vi "UHR-Fleezers Control (host) - 12.5.vi"() -> ()   [LabVIEW 2012] (continued)
    n2798 = xnode ("Read/Write Control")("FPGA VI Reference In"=w3268, "error in"=w3267) -> ("FPGA VI Reference Out"=w3103:T20, "error out"=w3102:errorcluster, "AI2 Y Sum Set 1"=w3366:i16, "AI2 Y Sum Set 2"=w3365:i16, "AI1 X Set 1"=w3167:fxp<+/-,16,1>, "AI1 X Set 2"=w3166:fxp<+/-,16,1>, "Trap Pos FB Int Signal"=→"Trap Pos FB Int Signal":fxp<+/-,24,9>, "Trap Pos FB Int-Norm Signal"=→"Trap Pos FB Int-Norm Signal":fxp<+/-,16,1>, "Trap Pos FB Action"=w3160:i64, "Scanning"=→"AOD Scanning":bool, "Scan I"=→"AOD Scan I":u64, "Scanning MCL"=w3368:bool, "Scan I (MCL)"=→"MCL Scan I":u64, "Green FB Sum"=w3305:i16, "Trap Pos FB Action"=w3090:i64, "TTrig Fin Thresh"=w3086:i64, "Red FB Intensity"=w3067:i16, "Blue Intensity"=w3062:i16)
    "MCL Scanning" <- w3368
    "Trap Pos FB Action" <- w3160
    n2799 = Divide(x=w3067, y=3276.7) -> (x/y=w3066:dbl)
    "Red laser intensity (V)" <- w3066
    n2800 = Divide(x=w3062, y=3276.7) -> (x/y=w3061:dbl)
    "Blue laser intensity (V)" <- w3061
    n2801 = Divide(x=w3305, y=3276.7) -> (x/y=w3065:dbl)
    "Green laser intensity (V)" <- w3065
    n2802 = local read "FB Trig Integrate"() -> (w3084:u32)
    n2803 = Divide(x=w3090, y=w3084) -> (x/y=w3083:dbl)
    "TTrig Sig (Int)" <- w3083
    n2804 = Bundle(w3065, w3066, w3061) -> (→"Fluorescence laser intensities plot":cluster{dbl, dbl, dbl})  [unwired: 1 in]
    n2805 = Divide(x=w3086, y=w3084) -> (x/y=w3081:dbl)
    "TTrig Fin Thresh (Int)" <- w3081
    n2806 = local read "AOM X Cal (nm/MHz)"() -> (w3089:dbl)
    n2807 = local read "AI2 (V)"() -> (w3367:cluster{"Set 1":dbl, "Set 2":dbl})
    n2808 = Bundle By Name(cluster=w3367, "Set 1"=w3366, "Set 2"=w3365) -> (w3363:cluster{"Set 1":dbl, "Set 2":dbl})
    n2809 = Divide(x=w3160, y=327.67) -> (x/y=→"Action (%)":dbl)
    n2810 = local read "Trap X (AI1)"() -> (w3180:T10)
    n2811 = call "IR AOM word double to freq.vi"("Frequency Word In (double)"=w3081) -> ("Frequency Out (MHz)"=w3080:dbl)
    n2812 = call "IR AOM word double to freq.vi"("Frequency Word In (double)"=w3083) -> ("Frequency Out (MHz)"=w3082:dbl)
    n2813 = Divide(x=w3363, y=3276.7) -> (x/y=w3362:cluster{"Set 1":dbl, "Set 2":dbl})
    n2814 = Multiply(x=w3082, y=w3089) -> (x*y=w3088:dbl)
    "TTrig Sig (nm)" <- w3088
    n2815 = Multiply(x=w3080, y=w3089) -> (x*y=w3087:dbl)
    "TTrig Fin Thresh (nm)" <- w3087
    n2816 = local write "AI2 (V)"(w3362) -> ()
    n2817 = Bundle(cluster=w3180, "Trap 1"=w3167, "Trap 2"=w3166) -> (→"Trap X (AI1)":T10)
    n2818 = Bundle(w3088, w3087) -> (→"TTrig":cluster{dbl, dbl})  [unwired: 1 in]
    n2819 = flat-sequence "To save data" {
      tunnel: [w4458] -> w3386
      tunnel: [w4459] -> w3385
      tunnel: w3336 -> [w4452]
      tunnel: w3108 -> [w4456]
      tunnel: ["Save Calibration"] -> w3359
      tunnel: w3356 -> [w4455]
      tunnel: [w4448] -> w3355
      tunnel: [w4445] -> w3354
      tunnel: [w4442] -> w3353
      tunnel: w3335 -> [w4444]
      tunnel: w3250 -> [w4438]
      tunnel: [w4438] -> w3249
      tunnel: ["Start Saving"] -> w3219
      tunnel: [w4432] -> w3148
      tunnel: [w4431] -> w3147
      tunnel: w3386 -> [w4706]
      tunnel: w3385 -> [w4705]
      tunnel: w3149 -> [w4704]
      tunnel: w3359 -> [w4703]
      tunnel: w3355 -> [w4701]
      tunnel: w3354 -> [w4700]
      tunnel: w3353 -> [w4699]
      tunnel: w3228 -> [w4698]
      tunnel: w3260 -> [w4697]
      tunnel: w3249 -> [w4696]
      tunnel: w3219 -> [w4695]
      tunnel: w3217 -> [w4694]
      tunnel: w3045 -> [w4693]
      tunnel: w3148 -> [w4692]
      tunnel: w3147 -> [w4691]
      tunnel: w3146 -> [w4690]
      tunnel: w3069 -> [w4689]
      frame #0 {
        n2820 = Or(x="Save N Sets", y="Start Saving") -> (x .or. y?=w4439:bool)
        n2821 = To Double Precision Float(number=w4455) -> (double precision float=w4449:dbl)
        n2822 = Build Array(w4439, "Save Calibration", w4452, w4444) -> (w4454:bool[])
        n2823 = Compound Arithmetic op=OR("Save Calibration", w4452, w4439, w4444) -> (w4457:bool)
        n2824 = Boolean Array To Number(Boolean array=w4454) -> (number=w4451:u32)
        n2825 = feedback #27(FALSE ("Save APD Data\nwith Trap Data")) -> (w4433:bool)
        n2826 = feedback #28(refnum<k0> refnum) -> (w4460:refnum<file>)
        n2827 = feedback #29(refnum<k0> refnum) -> (w4435:refnum<file>)
        n2828 = feedback #30(FALSE ("Save APD Data\nwith Trap Data")) -> (w4443:bool)
        n2829 = feedback #31(refnum<k0> refnum) -> (w4446:refnum<file>)
        n2830 = feedback #32(0) -> (w4462:i32)
        n2831 = feedback #33() -> (w4450:u32)  [unwired: 1 out]
        n2832 = case shown="True" w4457 {
          tunnel: [w4469 1] -> w4458
          tunnel: w4462 -> [w4471 _]
          tunnel: [w4470 w4502] -> w4459
          tunnel: w4460 -> [w4470 _]
          tunnel: w4456 -> [_ w4520]
          tunnel: w4449 -> [_ w4518]
          tunnel: w4451 -> [_ w4521]
          tunnel: [w4468 w4501] -> w4448
          tunnel: w4450 -> [w4468 _]
          tunnel: [w4467 w4499] -> w4445
          tunnel: w4446 -> [w4467 _]
          tunnel: [w4466 w4498] -> w4442
          tunnel: w4443 -> [w4466 _]
          tunnel: "Start Saving" -> [_ w4496]
          tunnel: w4438 -> [_ w4495]
          tunnel: [w4465 w4487] -> w4431
          tunnel: w4435 -> [w4465 _]
          tunnel: [w4464 w4486] -> w4432
          tunnel: w4433 -> [w4464 _]
          frame False {
            n2833 = Increment(x=w4471) -> (x+1=w4469:i32)
          }
          frame True {
            w4492 = FALSE ("Start Saving")
            w4497 = 9.0  # File Version
            w4504 = FALSE ("prepend array or string size? (T)")
            w4503 = T27."big-endian, network order" ("byte order (0:big-endian, network order)")
            n2834 = local read "BD 1 Frequency 1 (MHz)"() -> (w4517:dbl)
            n2835 = local read "BD 2 Frequency 1 (MHz)"() -> (w4516:dbl)
            n2836 = local read "BD 1 Frequency 2 (MHz)"() -> (w4515:dbl)
            n2837 = local read "BD 2 Frequency 2 (MHz)"() -> (w4514:dbl)
            n2838 = local read "BD 1 Frequency 3 (MHz)"() -> (w4513:dbl)
            n2839 = local read "BD 2 Frequency 3 (MHz)"() -> (w4512:dbl)
            n2840 = Array Size(array=w4495) -> (size(s)=w4494:i32)
            n2841 = To Double Precision Float(number=w4494) -> (double precision float=w4493:dbl)
            n2842 = local write "Save Calibration"(w4492) -> ()
            n2843 = local write "Start Saving"(w4492) -> ()
            n2844 = Build Array("Save APD Data\nwith Trap Data", "Save Trap Pos. Data") -> (w4489:bool[])
            n2845 = Boolean Array To Number(Boolean array=w4489) -> (number=w4488:u32)
            n2846 = Build Array(w4517, w4516, w4515, w4514, w4513, w4512) -> (w4511:dbl[])
            n2847 = case shown="1, Default" w4521 {
              tunnel: w4520 -> [w4593 w4613 w4629 w4667]
              tunnel: w4493 -> [w4598 w4620 w4649 w4686]
              tunnel: w4518 -> [w4597 w4619 w4648 w4685]
              tunnel: [w4594 w4615 w4640 w4677] -> w4509
              tunnel: [w4585 "Cal sets to save" w4630 w4668] -> w4501
              tunnel: w4511 -> [w4595 w4616 w4642 w4679]
              tunnel: "Save APD Data\nwith Trap Data" -> [w4592 _ w4626 w4665]
              tunnel: [w4592 w4607 w4626 w4665] -> w4498
              tunnel: w4497 -> [w4588 w4608 w4624 w4663]
              tunnel: w4496 -> [w4587 _ _ _]
              tunnel: [w4578 w4607 w4623 w4653] -> w4486
              tunnel: "Save Trap Pos. Data" -> [w4578 _ w4623 w4653]
              tunnel: w4488 -> [w4577 _ w4622 w4652]
              frame 1, Default {
                # "timeseries"
                n2848 = case shown="True" "Profile" {
                  tunnel: [w4601 w4605] -> w4582
                  tunnel: [w4601 w4604] -> w4581
                  tunnel: [w4601 w4603] -> w4580
                  tunnel: [w4601 w4602] -> w4579
                  frame False {
                    w4601 = 0.0 ("f")
                  }
                  frame True {
                    n2849 = local read "Current Position"() -> (w4606:cluster{dbl, dbl, dbl})
                    n2850 = local read "Y change (mm)"() -> (w4602:dbl)
                    n2851 = Unbundle(w4606) -> (w4605:dbl, w4604:dbl, w4603:dbl)
                  }
                }
                n2852 = local read "Save ave N"() -> (w4600:dbl)
                n2853 = Multiply(x=w4600, y=w4593) -> (x*y=w4599:dbl)
                n2854 = To Double Precision Float(number=w4577) -> (double precision float=w4591:dbl)
                n2855 = Build Array(w4588, w4593, w4599, w4598, w4597, 0.0 ("f")) -> (w4596:dbl[])
                n2856 = Build Array(w4591, w4582, w4581, w4580, w4579) -> (w4589:dbl[])
                n2857 = Select(t=u32 4000000000, s=w4587, f="N sets to save") -> (s? t:f=w4585:u32)
                n2858 = Build Array (concatenate)(w4596, w4595, w4589) -> (w4594:dbl[])
              }
              frame 2 {
                w4610 = 0.0 ("f")
                w4607 = FALSE ("Save APD Data\nwith Trap Data")
                # "calibration"
                n2859 = Boolean To (0,1)(Boolean=w4607) -> (0, 1=w4612:i16)
                n2860 = To Double Precision Float(number=w4612) -> (double precision float=w4611:dbl)
                n2861 = Build Array(w4611, w4610, w4610, w4610, w4610) -> (w4609:dbl[])
                n2862 = Build Array(w4608, w4613, w4613, w4620, w4619, 1.0 ("t")) -> (w4617:dbl[])
                n2863 = Build Array (concatenate)(w4617, w4616, w4609) -> (w4615:dbl[])
                "Calibrating Trap..." <- TRUE ("Calibrating...")
              }
              frame 4 {
                w4627 = 0.0 ("f")
                # "scan dir (x/y = 0/1)"
                # "cycles/step"
                # "n scans (f/b)"
                # "steps"
                # "freq. range"
                # "AOD raster scan"
                n2864 = local read "Number of F/B Scans (AOD)"() -> (w4634:u16)
                n2865 = local read "Cycles/step (AOD)"() -> (w4636:u64)
                n2866 = local read "Scan Range (MHz)"() -> (w4639:dbl)
                n2867 = local read "Scan steps (AOD)"() -> (w4638:u64)
                n2868 = local read "Scan BD"() -> (w4646:bool)
                n2869 = local read "Save ave N"() -> (w4651:dbl)
                n2870 = Boolean To (0,1)(Boolean=w4646) -> (0, 1=w4645:i16)
                n2871 = To Double Precision Float(number=w4634) -> (double precision float=w4633:dbl)
                n2872 = To Double Precision Float(number=w4638) -> (double precision float=w4637:dbl)
                n2873 = To Double Precision Float(number=w4636) -> (double precision float=w4635:dbl)
                n2874 = To Double Precision Float(number=w4645) -> (double precision float=w4644:dbl)
                n2875 = Multiply(x=w4651, y=w4629) -> (x*y=w4650:dbl)
                n2876 = To Double Precision Float(number=w4622) -> (double precision float=w4628:dbl)
                n2877 = Build Array(w4628, w4627, w4627, w4627, w4627) -> (w4625:dbl[])
                n2878 = local read "N sets should be saved"() -> (w4631:dbl)
                n2879 = Build Array(w4644, w4639, w4637, w4635, w4633) -> (w4641:dbl[])
                n2880 = Build Array(w4624, w4629, w4650, w4649, w4648, 2.0 ("t")) -> (w4643:dbl[])
                n2881 = Round Toward +Infinity(x=w4631) -> (ceil(x): smallest int >= x=w4632:dbl)
                n2882 = Build Array (concatenate)(w4643, w4642, w4625, w4641) -> (w4640:dbl[])
                n2883 = To Unsigned Long Integer(number=w4632) -> (unsigned 32bit integer=w4630:u32)
              }
              frame 8 {
                w4660 = 0.0 ("f")
                # "MCL raster scan"
                n2884 = local read "Number of scans (MCL)"() -> (w4655:u64)
                n2885 = local read "Scan lines (y)"() -> (w4654:u64)
                n2886 = local read "2D or 1D Scan"() -> (w4657:bool)
                n2887 = local read "Scan Range (V)\n(of steps)"() -> (w4676:dbl)
                n2888 = local read "Fast Scan Dir"() -> (w4683:bool)
                n2889 = local read "Cycles/step (MCL)"() -> (w4673:u64)
                n2890 = local read "Scan steps (MCL)"() -> (w4675:u64)
                n2891 = Select(t=w4654, s=w4657, f=w4655) -> (s? t:f=w4656:u64)
                n2892 = Boolean To (0,1)(Boolean=w4657) -> (0, 1=w4659:i16)
                n2893 = local read "Save ave N"() -> (w4688:dbl)
                n2894 = local read "Initial X"() -> (w4662:dbl)
                n2895 = local read "Initial Y"() -> (w4661:dbl)
                n2896 = To Double Precision Float(number=w4659) -> (double precision float=w4658:dbl)
                n2897 = Boolean To (0,1)(Boolean=w4683) -> (0, 1=w4682:i16)
                n2898 = To Double Precision Float(number=w4656) -> (double precision float=w4671:dbl)
                n2899 = To Double Precision Float(number=w4675) -> (double precision float=w4674:dbl)
                n2900 = To Double Precision Float(number=w4673) -> (double precision float=w4672:dbl)
                n2901 = To Double Precision Float(number=w4682) -> (double precision float=w4681:dbl)
                n2902 = Multiply(x=w4688, y=w4667) -> (x*y=w4687:dbl)
                n2903 = To Double Precision Float(number=w4652) -> (double precision float=w4666:dbl)
                n2904 = local read "N sets should be saved (MCL)"() -> (w4669:dbl)
                n2905 = Build Array(w4666, w4658, w4660, w4660, w4660) -> (w4664:dbl[])
                n2906 = Build Array(w4681, w4676, w4674, w4672, w4671, w4662, w4661) -> (w4678:dbl[])
                n2907 = Build Array(w4663, w4667, w4687, w4686, w4685, 3.0 ("t")) -> (w4680:dbl[])
                n2908 = Round Toward +Infinity(x=w4669) -> (ceil(x): smallest int >= x=w4670:dbl)
                n2909 = Build Array (concatenate)(w4680, w4679, w4664, w4678) -> (w4677:dbl[])
                n2910 = To Unsigned Long Integer(number=w4670) -> (unsigned 32bit integer=w4668:u32)
              }
            }
            n2911 = local read "Index"() -> (w4526:dbl)
            n2912 = call "Create new save file.vi"("Insert"="", "Ext"=".dat", "Index In"=w4526) -> ("Path Out"=w4482:path, "Index Out"=w4500:dbl)
            n2913 = local write "Save file name"(w4482) -> ()
            n2914 = local write "Index"(w4500) -> ()
            n2915 = local write "Save index"(w4500) -> ()
            n2916 = Array Size(array=w4509) -> (size(s)=w4510:i32)
            n2917 = Open/Create/Replace File(file path (use dialog)=w4482, operation (0:open)=T28."create", access (0:read/write)=enum16{"read/write", "read-only", "write-only"}."write-only") -> (refnum out=w4523:refnum<file>)  [unwired: 1 in, 4 out]
            n2918 = local write "Saving..."(TRUE ("Saving...")) -> ()
            n2919 = To Double Precision Float(number=w4510) -> (double precision float=w4508:dbl)
            n2920 = String Length(string="Comment (data description)") -> (length=w4507:i32)
            n2921 = To Double Precision Float(number=w4507) -> (double precision float=w4506:dbl)
            n2922 = Deny Access(7:w4523) -> (3:w4522:refnum<file>)  [unwired: 1 in, 2 out]
            n2923 = Build Array (concatenate)(w4508, w4509, w4506) -> (w4481:dbl[])
            n2924 = case "If fluorescence data to be saved" shown="True" w4498 {
              tunnel: w4482 -> [_ w4576]
              tunnel: [refnum<k0> refnum w4556] -> w4499
              frame False {
              }
              frame True {
                w4555 = 0.0
                n2925 = local read "APD Integration Time (s)"() -> (w4561:dbl)
                n2926 = local read "N APD Samp/step"() -> (w4554:dbl)
                n2927 = local read "Number of APDs"() -> (w4553:u8)
                n2928 = Path To String(path=w4576) -> (string=w4575:string)
                n2929 = String Length(string=w4575) -> (length=w4574:i32)
                n2930 = Subtract(x=w4574, y=4) -> (x-y=w4572:i32)
                n2931 = String Subset(string=w4575, length (rest)=w4572) -> (substring=w4571:string)  [unwired: 1 out]
                n2932 = Build Array(w4561, w4554, w4553, w4555, w4555, w4555, w4555, w4555) -> (w4558:dbl[])
                n2933 = Concatenate Strings(w4571, "_fl.dat" ("string")) -> (w4569:string)
                n2934 = Array Size(array=w4558) -> (size(s)=w4560:i32)
                n2935 = String To Path(string=w4569) -> (path=w4565:path)
                n2936 = Open/Create/Replace File(file path (use dialog)=w4565, operation (0:open)=T28."create", access (0:read/write)=enum16{"read/write", "read-only", "write-only"}."write-only") -> (refnum out=w4566:refnum<file>)  [unwired: 1 in, 4 out]
                n2937 = Deny Access(7:w4566) -> (3:w4562:refnum<file>)  [unwired: 1 in, 2 out]
                n2938 = To Double Precision Float(number=w4560) -> (double precision float=w4559:dbl)
                n2939 = Build Array (concatenate)(w4559, w4558) -> (w4557:dbl[])
                n2940 = Write to Binary File(file (use dialog)=w4562, data=w4557, 5:FALSE ("prepend array or string size? (T)"), 9:T27."big-endian, network order" ("byte order (0:big-endian, network order)")) -> (refnum out=w4556:refnum<file>)  [unwired: 1 in, 3 out]
              }
            }
            n2941 = case shown="True" w4486 {
              tunnel: w4482 -> [_ w4537]
              tunnel: [refnum<k0> refnum w4536] -> w4487
              frame False {
              }
              frame True {
                w4532 = 0.0 ("element")
                n2942 = Path To String(path=w4537) -> (string=w4551:string)
                n2943 = Build Array(w4532, w4532, w4532, w4532, w4532, w4532, w4532, w4532) -> (w4533:dbl[])
                n2944 = String Length(string=w4551) -> (length=w4550:i32)
                n2945 = Subtract(x=w4550, y=4) -> (x-y=w4548:i32)
                n2946 = Array Size(array=w4533) -> (size(s)=w4535:i32)
                n2947 = String Subset(string=w4551, length (rest)=w4548) -> (substring=w4547:string)  [unwired: 1 out]
                n2948 = To Double Precision Float(number=w4535) -> (double precision float=w4534:dbl)
                n2949 = Concatenate Strings(w4547, "_pos.dat" ("string")) -> (w4545:string)
                n2950 = Build Array (concatenate)(w4534, w4533) -> (w4531:dbl[])
                n2951 = String To Path(string=w4545) -> (path=w4541:path)
                n2952 = Open/Create/Replace File(file path (use dialog)=w4541, operation (0:open)=T28."create", access (0:read/write)=enum16{"read/write", "read-only", "write-only"}."write-only") -> (refnum out=w4542:refnum<file>)  [unwired: 1 in, 4 out]
                n2953 = Deny Access(7:w4542) -> (3:w4538:refnum<file>)  [unwired: 1 in, 2 out]
                n2954 = Write to Binary File(file (use dialog)=w4538, data=w4531, 5:FALSE ("prepend array or string size? (T)"), 9:T27."big-endian, network order" ("byte order (0:big-endian, network order)")) -> (refnum out=w4536:refnum<file>)  [unwired: 1 in, 3 out]
              }
            }
            n2955 = Write to Binary File(file (use dialog)=w4522, data=w4481, 5:w4504, 9:w4503) -> (refnum out=w4505:refnum<file>)  [unwired: 1 in, 3 out]
            n2956 = Write to Binary File(file (use dialog)=w4505, data="Comment (data description)", 5:w4504, 9:w4503) -> (refnum out=w4502:refnum<file>)  [unwired: 1 in, 3 out]
            n2957 = local read "connection reference"() -> (w4484:T17)
            n2958 = Bundle("Comment (data description)"="Comment (data description)", "Channel 1 Buffer"="Channel 1 Buffer", "Channel 2 Buffer"="Channel 2 Buffer", "Channel 3 Buffer"="Channel 3 Buffer", "Title"="Title", "DNA Construct"="DNA Construct", "Bead diameter"="Bead diameter", "Name"="Name") -> (w4472:T46)  [unwired: 1 in]
            n2959 = call "MattFileCreator-v9.vi"("Comments"=w4472, "Input Array"=w4481, "File path"=w4482, "table"="labview", "connection reference"=w4484) -> ("connection reference out"=w4483:T17)  [unwired: 5 in, 1 out]
            n2960 = local write "connection reference"(w4483) -> ()
          }
        }
        n2961 = feedback-in #27(w4432) -> ()
        n2962 = feedback-in #28(w4459) -> ()
        n2963 = feedback-in #29(w4431) -> ()
        n2964 = feedback-in #30(w4442) -> ()
        n2965 = feedback-in #31(w4445) -> ()
        n2966 = feedback-in #32(w4458) -> ()
        n2967 = feedback-in #33(w4448) -> ()
      }
      frame #1 {
        n2968 = local read "Saving..."() -> (w4702:bool)
        n2969 = case shown="True" w4702 {
          tunnel: w4706 -> [_ w4717]
          tunnel: w4705 -> [_ w4731]
          tunnel: w4704 -> [_ w4727]
          tunnel: w4703 -> [_ w4726]
          tunnel: w4701 -> [_ w4725]
          tunnel: w4700 -> [_ w4720]
          tunnel: w4699 -> [_ w4719]
          tunnel: w4698 -> [_ w4718]
          tunnel: w4697 -> [_ w4716]
          tunnel: w4696 -> [_ w4714]
          tunnel: w4695 -> [_ w4713]
          tunnel: w4694 -> [_ w4712]
          tunnel: w4693 -> [_ w4711]
          tunnel: w4692 -> [_ w4710]
          tunnel: w4691 -> [_ w4709]
          tunnel: w4690 -> [_ w4708]
          tunnel: w4689 -> [_ w4707]
          frame False {
          }
          frame True {
            n2970 = Multiply(x=w4717, y=w4716) -> (x*y=→"Time (s)":dbl)
            n2971 = Less Or Equal?(x=w4717, y=w4725) -> (x <= y?=w4729:bool)
            n2972 = Or(x="Stop Saving", y="Abort save 2") -> (x .or. y?=w4721:bool)
            n2973 = Not(x=w4721) -> (.not. x?=w4730:bool)
            n2974 = And(x=w4729, y=w4730) -> (x .and. y?=w4728:bool)
            n2975 = case shown="True" w4728 {
              tunnel: w4731 -> [w4738 w4829]
              tunnel: [0.0 w4832] -> w4724
              tunnel: w4717 -> [_ w4830]
              tunnel: w4725 -> [_ w4831]
              tunnel: w4727 -> [_ w4826]
              tunnel: w4726 -> [_ _]
              tunnel: w4720 -> [w4736 w4819]
              tunnel: w4719 -> [w4735 w4820]
              tunnel: w4718 -> [_ w4818]
              tunnel: w4714 -> [_ w4817]
              tunnel: w4713 -> [_ w4741]
              tunnel: w4712 -> [_ w4810]
              tunnel: w4711 -> [_ w4757]
              tunnel: w4710 -> [w4732 w4774]
              tunnel: w4709 -> [w4733 w4773]
              tunnel: w4708 -> [_ w4770]
              tunnel: w4707 -> [_ w4768]
              frame False {
                w4734 = FALSE
                n2976 = Close File(refnum=w4738) -> ()  [unwired: 1 in, 2 out]
                n2977 = case shown="True" w4735 {
                  tunnel: w4736 -> [_ w4740]
                  frame False {
                  }
                  frame True {
                    n2978 = Close File(refnum=w4740) -> ()  [unwired: 1 in, 2 out]
                  }
                }
                n2979 = case shown="True" w4732 {
                  tunnel: w4733 -> [_ w4739]
                  frame False {
                  }
                  frame True {
                    n2980 = Close File(refnum=w4739) -> ()  [unwired: 1 in, 2 out]
                  }
                }
                n2981 = local write "Raster Scanning..."(w4734) -> ()
                n2982 = local write "Calibrating Trap..."(w4734) -> ()
                n2983 = call <vilib>:"Beep.vi"() -> ()  [unwired: 3 in, 9 out]
                n2984 = local write "Stop Saving"(w4734) -> ()
                "Saving..." <- w4734
              }
              frame True {
                n2985 = local read "Calibrating Trap..."() -> (w4821:bool)
                n2986 = case "Write fl. data" shown="True" w4820 {
                  tunnel: w4819 -> [_ w4855]
                  tunnel: w4818 -> [_ w4854]
                  frame False {
                  }
                  frame True {
                    n2987 = Write to Binary File(file (use dialog)=w4855, data=w4854, 5:FALSE ("prepend array or string size? (T)"), 9:T27."big-endian, network order" ("byte order (0:big-endian, network order)")) -> ()  [unwired: 1 in, 4 out]
                  }
                }
                n2988 = Greater?(x="Save ave N", y=1.0) -> (0:w4824:bool)
                n2989 = Not(x=w4821) -> (.not. x?=w4823:bool)
                n2990 = And(x=w4823, y=w4824) -> (x .and. y?=w4771:bool)
                n2991 = case shown="True" w4771 {
                  tunnel: w4770 -> [w4835 w4846]
                  tunnel: [w4835 w4838] -> w4769
                  tunnel: "Save ave N" -> [_ w4839]
                  frame False {
                  }
                  frame True {
                    w4836 = 2 ("dimension size")
                    n2992 = Array Size(array=w4846) -> (size(s)=w4840:i32)
                    n2993 = Divide(x=w4840, y=w4836) -> (x/y=w4844:dbl)
                    n2994 = Reshape Array(w4846, w4844, w4836) -> (w4845:u64[][])
                    n2995 = Transpose 2D Array(2D array=w4845) -> (transposed array=w4843:u64[][])
                    n2996 = for {
                      tunnel: w4843 -> [w4848] mode=indexing
                      tunnel: [w4847] -> w4837 mode=indexing
                      tunnel: w4839 -> [w4849]
                      workers-P: _ -> [_]
                      n2997 = call "downsample 1D array - U64.vi"("Ave N"=w4849, "Array In"=w4848) -> ("Array Out"=w4847:u64[])  [unwired: 1 in]
                    }
                    n2998 = Transpose 2D Array(2D array=w4837) -> (transposed array=w4842:u64[][])
                    n2999 = Divide(x=w4840, y=w4839) -> (x/y=w4841:dbl)
                    n3000 = Reshape Array(w4842, w4841) -> (w4838:u64[])
                  }
                }
                n3001 = case shown="True" w4771 {
                  tunnel: w4826 -> [w4858 w4870]
                  tunnel: [w4858 w4862] -> w4822
                  tunnel: "Save ave N" -> [_ w4863]
                  tunnel: w4817 -> [_ w4861]
                  frame False {
                  }
                  frame True {
                    n3002 = Array Size(array=w4870) -> (size(s)=w4864:i32)
                    n3003 = Array Size(array=w4861) -> (size(s)=w4860:i32)
                    n3004 = Divide(x=w4864, y=w4860) -> (x/y=w4868:dbl)
                    n3005 = Reshape Array(w4870, w4868, w4860) -> (w4869:i16[][])
                    n3006 = Transpose 2D Array(2D array=w4869) -> (transposed array=w4867:i16[][])
                    n3007 = for {
                      tunnel: w4867 -> [w4873] mode=indexing
                      tunnel: [w4872] -> w4859 mode=indexing
                      tunnel: w4863 -> [w4871]
                      workers-P: _ -> [_]
                      n3008 = call "downsample 1D array - I16.vi"("Ave N"=w4871, "Array In"=w4873) -> ("Array Out"=w4872:i16[])  [unwired: 1 out]
                    }
                    n3009 = Transpose 2D Array(2D array=w4859) -> (transposed array=w4866:i16[][])
                    n3010 = Divide(x=w4864, y=w4863) -> (x/y=w4865:dbl)
                    n3011 = Reshape Array(w4866, w4865) -> (w4862:i16[])
                  }
                }
                n3012 = Index Array(array=w4757, index=2) -> (element=w4758:waveform(dbl))
                n3013 = Index Array(array=w4757, index=1) -> (element=w4791:waveform(dbl))
                n3014 = Index Array(array=w4757, index=0) -> (element=w4793:waveform(dbl))
                n3015 = Unbundle By Name(w4758) -> ("Y"=w4760:dbl[])
                n3016 = Unbundle By Name(w4791) -> ("Y"=w4795:dbl[])
                n3017 = Unbundle By Name(w4793) -> ("Y"=w4803:dbl[])
                n3018 = case "Write trap pos. data" shown="True" w4774 {
                  tunnel: w4773 -> [_ w4851]
                  tunnel: w4769 -> [_ w4850]
                  frame False {
                  }
                  frame True {
                    n3019 = Write to Binary File(file (use dialog)=w4851, data=w4850, 5:FALSE ("prepend array or string size? (T)"), 9:T27."big-endian, network order" ("byte order (0:big-endian, network order)")) -> ()  [unwired: 1 in, 4 out]
                  }
                }
                n3020 = Write to Binary File(file (use dialog)=w4829, data=w4822, 5:FALSE ("prepend array or string size? (T)"), 9:T27."big-endian, network order" ("byte order (0:big-endian, network order)")) -> ()  [unwired: 1 in, 4 out]
                n3021 = feedback #34(w4760) -> (w4761:dbl[])
                n3022 = Build Array (concatenate)(w4761, w4760) -> (w4756:dbl[])
                n3023 = Select(t=w4760, s=w4741, f=w4756) -> (s? t:f=w4746:dbl[])
                n3024 = feedback-in #34(w4746) -> ()
                n3025 = feedback #35(w4795) -> (w4797:dbl[])
                n3026 = Build Array (concatenate)(w4797, w4795) -> (w4796:dbl[])
                n3027 = Select(t=w4795, s=w4741, f=w4796) -> (s? t:f=w4785:dbl[])
                n3028 = feedback-in #35(w4785) -> ()
                n3029 = feedback #36(w4803) -> (w4816:dbl[])
                n3030 = Build Array (concatenate)(w4816, w4803) -> (w4815:dbl[])
                n3031 = Select(t=w4803, s=w4741, f=w4815) -> (s? t:f=w4790:dbl[])
                n3032 = feedback-in #36(w4790) -> ()
                n3033 = Divide(x=w4830, y=w4831) -> (x/y=w4833:dbl)
                n3034 = Multiply(x=w4833, y=100.0) -> (x*y=w4832:dbl)
                n3035 = Build Array(w4790, w4785, w4746) -> (→"Saved APD":dbl[][])
                n3036 = Array Size(array=w4790) -> (size(s)=w4808:i32)
                n3037 = Unbundle By Name(w4810) -> ("Y"=w4814:dbl[])
                n3038 = Subtract(x=w4808, y="N pts to average") -> (x-y=w4743:i32)
                n3039 = Multiply(x="N pts to average", y=u16 2) -> (x*y=w4786:u16)
                n3040 = Subtract(x=w4808, y=w4786) -> (x-y=w4744:i32)
                n3041 = feedback #37(w4814) -> (w4813:dbl[])
                n3042 = Build Array (concatenate)(w4813, w4814) -> (w4812:dbl[])
                n3043 = Select(t=w4814, s=w4741, f=w4812) -> (s? t:f=w4811:dbl[])
                "Trap Delta Graph" <- w4811
                n3044 = feedback-in #37(w4811) -> ()
                n3045 = Array Subset(array=w4790, index=w4743, length="N pts to average") -> (w4807:dbl[])
                n3046 = Array Subset(array=w4790, index=w4744, length="N pts to average") -> (w4806:dbl[])
                n3047 = Array Subset(array=w4785, index=w4743, length="N pts to average") -> (w4788:dbl[])
                n3048 = Array Subset(array=w4785, index=w4744, length="N pts to average") -> (w4787:dbl[])
                n3049 = Array Subset(array=w4746, index=w4743, length="N pts to average") -> (w4755:dbl[])
                n3050 = Array Subset(array=w4746, index=w4744, length="N pts to average") -> (w4754:dbl[])
                n3051 = Index Array(array=w4768, index=0) -> (element=w4766:waveform(dbl))
                n3052 = call-poly <vilib>:"Mean.vi"("X"=w4807) -> ("mean"=w4805:dbl)  [unwired: 1 out]
                n3053 = call-poly <vilib>:"Mean.vi"("X"=w4788) -> ("mean"=w4784:dbl)  [unwired: 1 out]
                n3054 = call-poly <vilib>:"Mean.vi"("X"=w4806) -> ("mean"=w4804:dbl)  [unwired: 1 out]
                n3055 = call-poly <vilib>:"Mean.vi"("X"=w4787) -> ("mean"=w4783:dbl)  [unwired: 1 out]
                n3056 = call-poly <vilib>:"Mean.vi"("X"=w4755) -> ("mean"=w4753:dbl)  [unwired: 1 out]
                n3057 = call-poly <vilib>:"Mean.vi"("X"=w4754) -> ("mean"=w4752:dbl)  [unwired: 1 out]
                n3058 = Unbundle By Name(w4766) -> ("Y"=w4764:dbl[])
                n3059 = Subtract(x=w4784, y=w4783) -> (x-y=w4775:dbl)
                "Delta Fl. 2" <- w4775
                n3060 = Subtract(x=w4753, y=w4752) -> (x-y=w4747:dbl)
                "Delta Fl. 3" <- w4747
                n3061 = Subtract(x=w4805, y=w4804) -> (x-y=w4802:dbl)
                "Delta Fl. 1" <- w4802
                n3062 = feedback #38(w4764) -> (w4763:dbl[])
                n3063 = Build Array (concatenate)(w4763, w4764) -> (w4765:dbl[])
                n3064 = Initialize Array(w4802, 1 ("dimension size")) -> (w4799:dbl[])
                n3065 = Initialize Array(w4775, 1 ("dimension size")) -> (w4780:dbl[])
                n3066 = Initialize Array(w4747, 1 ("dimension size")) -> (w4749:dbl[])
                n3067 = Select(t=w4764, s=w4741, f=w4765) -> (s? t:f=w4762:dbl[])
                "Saved trap pos" <- w4762
                n3068 = feedback-in #38(w4762) -> ()
                n3069 = feedback #39(w4799) -> (w4800:dbl[])
                n3070 = Build Array (concatenate)(w4800, w4799) -> (w4798:dbl[])
                n3071 = feedback #40(w4780) -> (w4781:dbl[])
                n3072 = feedback #41(w4749) -> (w4750:dbl[])
                n3073 = Build Array (concatenate)(w4781, w4780) -> (w4779:dbl[])
                n3074 = Build Array (concatenate)(w4750, w4749) -> (w4748:dbl[])
                n3075 = Select(t=w4799, s=w4741, f=w4798) -> (s? t:f=w4778:dbl[])
                n3076 = feedback-in #39(w4778) -> ()
                n3077 = Select(t=w4780, s=w4741, f=w4779) -> (s? t:f=w4777:dbl[])
                n3078 = feedback-in #40(w4777) -> ()
                n3079 = Select(t=w4749, s=w4741, f=w4748) -> (s? t:f=w4742:dbl[])
                n3080 = feedback-in #41(w4742) -> ()
                n3081 = Build Array(w4778, w4777, w4742) -> (→"Save APD Deriv":dbl[][])
              }
            }
            "Progress" <- w4724
            "Progress 2" <- w4724
          }
        }
      }
    }
    n3082 = local read "wait to reset values"() -> (w3370:bool)
    n3083 = Not(x=w3368) -> (.not. x?=w3371:bool)
    n3084 = And(x=w3371, y=w3370) -> (x .and. y?=w3372:bool)
    n3085 = case "Part of MCL raster scanning: returns to initial positions after scan done" shown="True" w3372 {
      tunnel: w3103 -> [w4252 w4259]
      tunnel: [w4252 w4258] -> w3374
      tunnel: w3102 -> [w4251 w4257]
      tunnel: [w4251 w4256] -> w3369
      frame False {
      }
      frame True {
        w4267 = 10.0 ("y")
        w4266 = 32767.0 ("y")
        # "to return scan values\nafter a synchronous \nAOM scan"
        n3086 = local read "AO2"() -> (w4260:dbl)
        n3087 = local read "AO1"() -> (w4261:dbl)
        n3088 = local write "wait to reset values"(FALSE ("wait to reset values")) -> ()
        n3089 = Multiply(x=w4261, y=w4266) -> (x*y=w4263:dbl)
        n3090 = Multiply(x=w4260, y=w4266) -> (x*y=w4265:dbl)
        n3091 = Divide(x=w4263, y=w4267) -> (x/y=w4262:dbl)
        n3092 = Divide(x=w4265, y=w4267) -> (x/y=w4264:dbl)
        n3093 = To Word Integer(number=w4262) -> (16bit integer=w4268:i16)
        n3094 = To Word Integer(number=w4264) -> (16bit integer=w4269:i16)
        n3095 = local read "Total Counts (ticks)"() -> (w4253:u16)
        n3096 = xnode "Read/Write Control"("FPGA VI Reference In"=w4259, "error in"=w4257, "AO1"=w4268, "AO2"=w4269, "MCL count"=w4253) -> ("FPGA VI Reference Out"=w4258:T20, "error out"=w4256:errorcluster)
        n3097 = local read "Scan Range (V)\n(of steps)"() -> (w4254:dbl)
        n3098 = property on="Scan Range (V)\n(of steps)" class="DigNum (strict)"("Val(Sgnl)"=w4254) -> ()  [unwired: 2 in, 2 out]
      }
    }
    n3099 = node-c288() -> ()  [unwired: 2 out]
  }
  n3100 = flat-sequence "Video" {
    tunnel: [w4883] -> w115
    tunnel: w115 -> [w4923]
    frame #0 {
      n3101 = while {
        stop <- w4875 continue-if-true
        n3102 = call "Close Video Capture.vi"() -> ("error code OUT"=w4877:i32)
        n3103 = Equal?(x=w4877, y=0) -> (x = y?=w4875:bool)
      }
      n3104 = local write "Stop All"(FALSE ("Stop All")) -> ()
    }
    frame #1 {
      n3105 = call "DMR_Init.vi"() -> ()  [unwired: 3 out]
    }
    frame #2 {
      w4878 = "DE245428202"  # MSU fleezers card #
      (unwired) "DE019116701"  # Illinois fleezers card #
      # "Setting the destination format to Mono8 makes sure that the image can be displayed in the intensity plot."
      n3106 = call "DMR_GetDevice.vi"("search string IN"=w4878) -> ("device handle OUT"=w4901:i32)  [unwired: 4 in, 2 out]
      n3107 = call "DMR_OpenDevice.vi"("device handle IN"=w4901) -> ("driver handle OUT"=w4884:i32)  [unwired: 4 out]
      n3108 = call "DMR_FindList.vi"("flags IN"=u32 0 ("flags"), "list name IN"="" ("String"), "list type IN"=T47."camera descriptions", "driver handle IN"=w4884) -> ("list handle OUT"=w4887:i32)  [unwired: 2 out]
      n3109 = call "DMR_FindList.vi"("flags IN"=u32 0 ("flags"), "list name IN"="Base", "list type IN"=T47."setting", "driver handle IN"=w4884) -> ("list handle OUT"=w4885:i32)  [unwired: 2 out]
      n3110 = call "OBJ_GetHandle.vi"("object name IN"="VideoStandard", "list handle IN"=w4887) -> ("object handle OUT"=w4881:i32)  [unwired: 3 out]
      n3111 = call "OBJ_GetHandle.vi"("object name IN"="PixelFormat", "list handle IN"=w4885) -> ("object handle OUT"=w4895:i32)  [unwired: 3 out]
      n3112 = call "OBJ_SetS.vi"("value index IN"=0, "value IN"="NTSC M", "object handle IN"=w4881) -> ()  [unwired: 2 out]
      n3113 = call "OBJ_SetS.vi"("value index IN"=0, "value IN"="Mono8" ("value"), "object handle IN"=w4895) -> ()  [unwired: 2 out]
      n3114 = call "OBJ_GetHandle.vi"("object name IN"="VideoChannel", "list handle IN"=w4885) -> ("object handle OUT"=w4891:i32)  [unwired: 3 out]
      n3115 = while {
        tunnel: [w4905] -> w4883
        tunnel: w4884 -> [w4902]
        stop <- w4903 continue-if-true
        n3116 = call "DMR_ImageRequestSingle.vi"("request control IN"=0, "driver handle IN"=w4902) -> ("error code OUT"=w4904:i32, "driver handle OUT"=w4905:i32)  [unwired: 2 out]
        n3117 = Equal To 0?(x=w4904) -> (x = 0?=w4903:bool)
      }
      n3118 = call "OBJ_SetI.vi"("value index IN"=0, "value IN"=3 ("Video channel"), "object handle IN"=w4891) -> ()  [unwired: 2 out]
    }
    frame #3 {
      w4911 = T18 0 items=["Grayscale (U8)", "Grayscale (I16)", "Grayscale (SGL)", "Complex (CSG)", "RGB (U32)", "HSL (U32)", "RGB (U64)"] ("Image Type")
      w4919 = T18 0 items=["Grayscale (U8)", "Grayscale (I16)", "Grayscale (SGL)", "Complex (CSG)", "RGB (U32)", "HSL (U32)", "RGB (U64)"] ("Image Type")
      n3119 = for "Create Greyscale map" {
        N: 256 -> [_]
        tunnel: [w4925] -> w4908 mode=indexing
        workers-P: _ -> [_]
        i -> [w4928]
        n3120 = To Unsigned Byte Integer(number=w4928) -> (unsigned 8bit integer=w4924:u8)
        n3121 = Join Numbers(hi=w4924, lo=w4924) -> ((hi.lo)=w4927:u16)
        n3122 = Join Numbers(hi=w4924, lo=w4924) -> ((hi.lo)=w4926:u16)
        n3123 = Join Numbers(hi=w4927, lo=w4926) -> ((hi.lo)=w4925:u32)
      }
      n3124 = call "IMAQ Create"("Image Name"="Scaled video", "Image Type"=w4911) -> ("New Image"=w4910:T2)  [unwired: 2 in, 2 out]
      n3125 = call "IMAQ Create"("Image Name"="Main video", "Image Type"=w4919) -> ("New Image"=w4920:T2)  [unwired: 2 in, 2 out]
      n3126 = node-c288(0 ("Processor")) -> (w4918:T23)  [unwired: 3 out]
      n3127 = Initialize Array(u32 0 ("Window Number (0...15)"), 480 ("dimension size"), 640 ("dimension size")) -> (w4913:u32[][])
      n3128 = timed-loop {
        tunnel: w4923 -> [w4945]
        tunnel: [w4944] -> w4922
        tunnel: w4920 -> [w4943]
        timing: w4918 -> [_]
        timing-out: [_] -> w4917
        tunnel: w4913 -> [w4932]
        tunnel: w4910 -> [w4930]
        tunnel: w4908 -> [w4929]
        stop <- w4931 stop-if-true
        # "This block performs the \nactual image capture."
        n3129 = node-c288() -> ()  [unwired: 2 out]
        n3130 = local read "Stop All"() -> (w4931:bool)
        n3131 = Reciprocal(x="Video Capture Rate (Hz)") -> (1/x=w4935:dbl)
        n3132 = Multiply(x=w4935, y=1000.0) -> (x*y=w4933:dbl)
        n3133 = call "DMR_ImageRequestWaitFor.vi"("queue number IN"=0, "timeout(ms) IN"=500, "driver handle IN"=w4945) -> ("error code OUT"=w4949:i32, "request number OUT"=w4946:i32, "driver handle OUT"=w4947:i32)
        n3134 = feedback #42(T48 refnum ("Avi Refnum")) -> (w4937:T48)
        n3135 = case shown="True" "New Video File" {
          tunnel: [T48 refnum ("Avi Refnum") w4966] -> w4939
          tunnel: [FALSE TRUE] -> w4940
          tunnel: w4937 -> [_ w4962]
          frame False {
          }
          frame True {
            n3136 = call "Create new save file.vi"("Ext"=".avi" ("string"), "Index In"="Video Index") -> ("Path Out"=w4958:path, "Index Out"=w4959:dbl)  [unwired: 1 in]
            "Path Out" <- w4958
            n3137 = Not Equal?(x=w4962, y=T48 refnum ("Avi Refnum")) -> (x != y?=w4963:bool)
            n3138 = Increment(x=w4959) -> (x+1=w4968:dbl)
            n3139 = case shown="True" w4963 {
              tunnel: w4962 -> [_ w4969]
              frame False {
              }
              frame True {
                n3140 = call "IMAQ AVI Close"("Avi Refnum"=w4969) -> ()  [unwired: 1 in, 10 out]
              }
            }
            n3141 = local write "Video Index"(w4968) -> ()
            n3142 = call "IMAQ AVI Create"("Frames Per Second"=u32 30, "AVI Path"=w4958) -> ("Avi Refnum"=w4966:T48)  [unwired: 5 in, 4 out]
          }
        }
        n3143 = Equal To 0?(x=w4949) -> (x = 0?=w4948:bool)
        n3144 = Select(t=w4939, s=w4940, f=w4937) -> (s? t:f=w4938:T48)
        n3145 = feedback-in #42(w4938) -> ()
        n3146 = case shown="True" w4948 {
          tunnel: w4947 -> [w4970 w5004]
          tunnel: w4946 -> [_ w5003]
          tunnel: [w4970 w5000] -> w4944
          tunnel: w4943 -> [_ w4985]
          tunnel: w4932 -> [_ w4989]
          tunnel: w4938 -> [_ w4987]
          tunnel: w4930 -> [_ w4982]
          tunnel: w4929 -> [_ w4981]
          frame False {
          }
          frame True {
            w4994 = u32 0 ("X-offset IN")
            n3147 = call "DMR_GetImageRequestBufferData.vi"("driver handle IN"=w5004, "request number IN"=w5003) -> ("width OUT"=w4993:i32, "height OUT"=w4992:i32, "driver handle OUT"=w4999:i32, "request number OUT"=w4998:i32, "bytes per pixel OUT"=w4995:i32)  [unwired: 13 out]
            n3148 = call "DMR_GetImageRequestBufferImageData.vi"("driver handle IN"=w4999, "request number IN"=w4998, "bytes per pixel IN"=w4995, "X-offset IN"=w4994, "Y-offset IN"=w4994, "height IN"=w4992, "width IN"=w4993) -> ("driver handle OUT"=w4997:u32, "request number OUT"=w4996:u32, "image OUT"=w4974:u32[][])  [unwired: 10 out]
            n3149 = Transpose 2D Array(2D array=w4974) -> (transposed array=w4980:u32[][])
            n3150 = Select(t=w4980, s="Flip Y (or X)", f=w4974) -> (s? t:f=w4979:u32[][])
            n3151 = call "DMR_ImageRequestUnlock.vi"("request number IN"=w4996, "driver handle IN"=w4997) -> ("driver handle OUT"=w5002:i32)  [unwired: 1 in, 2 out]
            n3152 = for {
              tunnel: w4979 -> [w5039] mode=indexing
              tunnel: [w5038] -> w4977 mode=indexing
              n3153 = Reverse 1D Array(array=w5039) -> (reversed array=w5038:u32[])
            }
            n3154 = call "DMR_ImageRequestSingle.vi"("request control IN"=0, "driver handle IN"=w5002) -> ("driver handle OUT"=w5000:i32)  [unwired: 3 out]
            n3155 = Transpose 2D Array(2D array=w4977) -> (transposed array=w4978:u32[][])
            n3156 = Select(t=w4978, s="Flip Y (or X)", f=w4977) -> (s? t:f=w4975:u32[][])
            n3157 = Select(t=w4975, s="Flip Image", f=w4974) -> (s? t:f=w4972:u32[][])
            n3158 = case shown="True" "Averaging" {
              tunnel: w4972 -> [w5042 w5047]
              tunnel: [w5042 w5046] -> w4986
              tunnel: w4989 -> [_ w5044]
              frame False {
              }
              frame True {
                (unwired) 1
                w5052 = 1
                n3159 = feedback #43(w5044) -> (w5043:u32[][])
                n3160 = Add(x=w5047, y=w5043) -> (x+y=w5048:u32[][])
                n3161 = Select(t=w5044, s="Reset Averaging", f=w5048) -> (s? t:f=w5050:u32[][])
                n3162 = feedback-in #43(w5050) -> ()
                n3163 = feedback #44(w5052) -> (w5045:i32)
                n3164 = Divide(x=w5048, y=w5045) -> (x/y=w5049:dbl[][])
                n3165 = Increment(x=w5045) -> (x+1=w5053:i32)
                n3166 = To Unsigned Long Integer(number=w5049) -> (unsigned 32bit integer=w5046:u32[][])
                n3167 = Select(t=w5052, s="Reset Averaging", f=w5053) -> (s? t:f=w5051:i32)
                n3168 = feedback-in #44(w5051) -> ()
              }
            }
            n3169 = case shown="True" "Zoom video window" {
              tunnel: w4986 -> [_ w5018]
              tunnel: w4982 -> [_ w5017]
              frame False {
              }
              frame True {
                n3170 = To Double Precision Float(number=w5018) -> (double precision float=w5015:dbl[][])
                n3171 = In Range and Coerce(upper limit="Intensity Upper", x=w5015, lower limit="Intensity Lower") -> (coerced(x)=w5014:dbl[][])  [unwired: 1 out]
                n3172 = Subtract(x="Intensity Upper", y="Intensity Lower") -> (x-y=w5011:dbl)
                n3173 = Subtract(x=w5014, y="Intensity Lower") -> (x-y=w5012:dbl[][])
                n3174 = Divide(x=w5012, y=w5011) -> (x/y=w5013:dbl[][])
                n3175 = Multiply(x=255.0, y=w5013) -> (x*y=w5009:dbl[][])
                n3176 = To Unsigned Byte Integer(number=w5009) -> (unsigned 8bit integer=w5016:u8[][])
                n3177 = call "IMAQ ArrayToImage"("Image Pixels (U8)"=w5016, "Image"=w5017) -> ("Image Out"=w5005:T2)  [unwired: 4 in, 5 out]
                n3178 = First Call?() -> (First Call?: T/F=w5006:bool)
                n3179 = case shown="True" w5006 {
                  tunnel: w5005 -> [w5019 w5030]
                  frame False {
                    n3180 = flat-sequence {
                      tunnel: w5019 -> [w5025]
                      frame #0 {
                        w5022 = FALSE ("Get/Set Status? (Set)")
                        w5021 = 0 ("Window Number (0...15)")
                        n3181 = call "IMAQ WindSize"("Get/Set Status? (Set)"=w5022, "Window Number"=w5021) -> ("Width & Height out"=→"Window Size":cluster{"Width":i32, "Height":i32})  [unwired: 4 in, 2 out]
                        n3182 = call "IMAQ WindMove"("Window Number (0...15)"=w5021, "Get/Set Status? (Set)"=w5022) -> ("Coordinates (screen)"=→"Window Position":cluster{"X Position":i32, "Y Position":i32})  [unwired: 3 in, 1 out]
                        n3183 = call "IMAQ WindDraw"("Resize to Image Size? (Y)"=FALSE, "Window Number (0...15)"=w5021, "Image"=w5025) -> ()  [unwired: 7 in, 2 out]
                      }
                      frame #1 {
                        n3184 = call "IMAQ WindZoom 2"("Center Point"="Center Point", "Zoom to Fit? (False)"=FALSE, "Zoom Factor"="Zoom Factor") -> ()  [unwired: 5 in, 4 out]
                      }
                    }
                  }
                  frame True {
                    n3185 = flat-sequence {
                      tunnel: w5030 -> [w5033]
                      tunnel: [w5031] -> w5029
                      tunnel: w5029 -> [w5035]
                      frame #0 {
                        w5032 = TRUE ("Resize to Image Size? (Y)")
                        w5031 = 0 ("Window Number (0...15)")
                        n3186 = call "IMAQ WindNonTearing"("Window Number"=w5031, "NonTearing? (True)"=w5032) -> ()  [unwired: 8 in, 2 out]
                        n3187 = call "IMAQ WindDraw"("Resize to Image Size? (Y)"=w5032, "Window Number (0...15)"=w5031, "Image"=w5033) -> ()  [unwired: 7 in, 2 out]
                      }
                      frame #1 {
                        n3188 = call "IMAQ WindSize"("Scrollbars? (N)"=FALSE, "Width & Height"="Initial Window Size", "Window Number"=w5035) -> ()  [unwired: 3 in, 3 out]
                        n3189 = call "IMAQ WindMove"("Window Number (0...15)"=w5035, "Coordinates (screen)"="Initial Window Position") -> ()  [unwired: 3 in, 2 out]
                      }
                    }
                  }
                }
              }
            }
            n3190 = To Unsigned Byte Integer(number=w4986) -> (unsigned 8bit integer=w4984:u8[][])
            n3191 = call "IMAQ ArrayToImage"("Image Pixels (U8)"=w4984, "Image"=w4985) -> ("Image Out"=w4983:T2)  [unwired: 4 in, 5 out]
            "Primary Video Display" <- w4983
            n3192 = case shown="True" "Save Video" {
              tunnel: w4987 -> [_ w5041]
              tunnel: w4983 -> [_ w5040]
              frame False {
              }
              frame True {
                n3193 = call "IMAQ AVI Write Frame"("Image"=w5040, "Avi Refnum"=w5041) -> ()  [unwired: 2 in, 8 out]
              }
            }
            n3194 = case shown="True" "Save Image" {
              tunnel: w4984 -> [_ w5056]
              tunnel: w4981 -> [_ w5055]
              frame False {
              }
              frame True {
                n3195 = call <vilib>:"Flatten Pixmap.vi"("colors"=w5055, "8-bit pixmap"=w5056) -> ("image data"=w5062:T49)  [unwired: 4 in, 5 out]
                n3196 = call "Create new save file.vi"("Insert"="video_frame_" ("string"), "Ext"=".bmp" ("string"), "Index In"="Image Index") -> ("Path Out"=w5058:path, "Index Out"=w5063:dbl)
                n3197 = Increment(x=w5063) -> (x+1=w5057:dbl)
                n3198 = local write "Image Index"(w5057) -> ()
                n3199 = call <vilib>:"Write BMP File.vi"("image data"=w5062, "path to BMP file"=w5058) -> ()  [unwired: 1 in, 9 out]
              }
            }
          }
        }
        n3200 = node-c288(w4933) -> ()  [unwired: 1 out]
      }
      n3201 = node-c288(w4917) -> ()  [unwired: 1 out]
      n3202 = call "DMR_CloseDevice.vi"("driver handle IN"=w4922) -> ()  [unwired: 1 in, 4 out]
    }
    frame #4 {
      n3203 = call "DMR_Close.vi"() -> ()  [unwired: 1 out]
    }
  }
  n3204 = timed-loop "Rough control of MCL mirror stage (debugging)" {
    tunnel: w13 -> [w5070]
    tunnel: [w5069] -> w255
    timing: w7 -> [_]
    timing-out: [_] -> w6
    stop <- w5069 stop-if-true
    n3205 = node-c288() -> ()  [unwired: 2 out]
    n3206 = case shown="1" "MCL Mode" {
      tunnel: w5070 -> [_ w5073 w5120]
      frame 0, Default {
      }
      frame 1 {
        n3207 = node-c288() -> (w5075:T23)  [unwired: 4 out]
        n3208 = timed-loop "Oscillate MCL mirror" {
          timing: w5075 -> [_]
          timing-out: [_] -> w5074
          tunnel: w5073 -> [w5114]
          i -> [w5113]
          stop <- w5076 stop-if-true
          n3209 = node-c288() -> (w5112:i64)  [unwired: 1 out]
          n3210 = Multiply(x="AO1", y=32767.0) -> (x*y=w5108:dbl)
          n3211 = Multiply(x="AO2", y=32767.0) -> (x*y=w5103:dbl)
          n3212 = Divide(x=w5108, y=10.0) -> (x/y=w5109:dbl)
          n3213 = Divide(x=w5103, y=10.0) -> (x/y=w5104:dbl)
          n3214 = To Word Integer(number=w5109) -> (16bit integer=w5101:i16)
          n3215 = To Word Integer(number=w5104) -> (16bit integer=w5100:i16)
          n3216 = Divide(x=w5112, y=i64 1000) -> (x/y=w5083:dbl)
          n3217 = Multiply(x=w5083, y=w5113) -> (x*y=w5094:dbl)
          n3218 = Multiply(x="Osc. freq. (Hz) 2", y=6.283185307179586) -> (x*y=w5095:dbl)
          n3219 = Multiply(x=w5095, y=w5094) -> (x*y=w5093:dbl)
          n3220 = Sine(x=w5093) -> (sin(x)=w5092:dbl)
          n3221 = Multiply(x=w5092, y="Osc. amp. (V)") -> (x*y=w5090:dbl)
          n3222 = Add(x=w5090, y="Osc. center (V)") -> (x+y=w5088:dbl)
          n3223 = Divide(x=w5088, y=10.0) -> (x/y=w5086:dbl)
          n3224 = Multiply(x=w5086, y=32767.0) -> (x*y=w5081:dbl)
          n3225 = Select(t=w5081, s="Scan axis", f=w5101) -> (s? t:f=w5099:dbl)
          n3226 = Select(t=w5100, s="Scan axis", f=w5081) -> (s? t:f=w5098:dbl)
          n3227 = local read "MCL Mode"() -> (w5080:u16)
          n3228 = Not Equal?(x=w5080, y=u16 1) -> (x != y?=w5077:bool)
          n3229 = local read "Stop All"() -> (w5078:bool)
          n3230 = xnode "Read/Write Control"("FPGA VI Reference In"=w5114, "AO1"=w5099, "AO2"=w5098) -> ()  [unwired: 1 in, 2 out]
          n3231 = Compound Arithmetic op=OR(w5078, w5077) -> (w5076:bool)
          n3232 = node-c288() -> ()  [unwired: 2 out]
        }
        n3233 = node-c288(w5074) -> ()  [unwired: 1 out]
      }
      frame 2 {
        n3234 = case shown="True" "Start Scan" {
          tunnel: w5120 -> [_ w5132]
          frame False {
          }
          frame True {
            n3235 = Subtract(x="End (V)", y="Begin (V)") -> (x-y=w5128:dbl)
            n3236 = Decrement(x="N Points") -> (x-1=w5127:dbl)
            n3237 = Divide(x=w5128, y=w5127) -> (x/y=w5125:dbl)
            n3238 = for {
              N: "N Points" -> [_]
              tunnel: "Begin (V)" -> [w5145]
              tunnel: w5132 -> [w5137]
              tunnel: [w5136] -> w5131 mode=indexing
              tunnel: w5125 -> [w5135]
              tunnel: [w5133] -> w5124 mode=indexing
              i -> [w5144]
              n3239 = Multiply(x=w5135, y=w5144) -> (x*y=w5143:dbl)
              n3240 = Add(x=w5145, y=w5143) -> (x+y=w5140:dbl)
              n3241 = local read "Scan axis"() -> (w5134:bool)
              n3242 = local read "AO1"() -> (w5142:dbl)
              n3243 = local read "AO2"() -> (w5141:dbl)
